vi "Exchange Tool.vi"(8 "error in":errorcluster, 9 "Tool Position":i32, 10 "Place/Pick":enum16{"Place", "Pick"}(ring), 11 "Gantry in":refnum<class "Gantry.lvclass">) -> (0 "error out":errorcluster, 3 "Gantry out":refnum<class "Gantry.lvclass">)   [LabVIEW 2017, in "Gantry.lvclass"]
uses:
  Gantry.lvclass
  Vec3d Class/Vec3d.lvclass
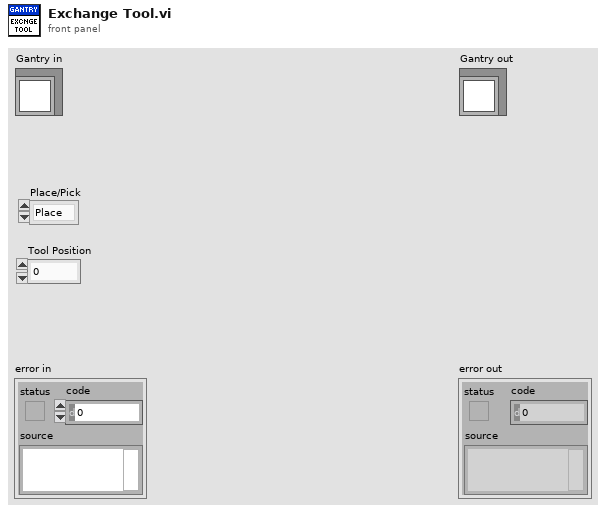
[diagram p1: front panel]
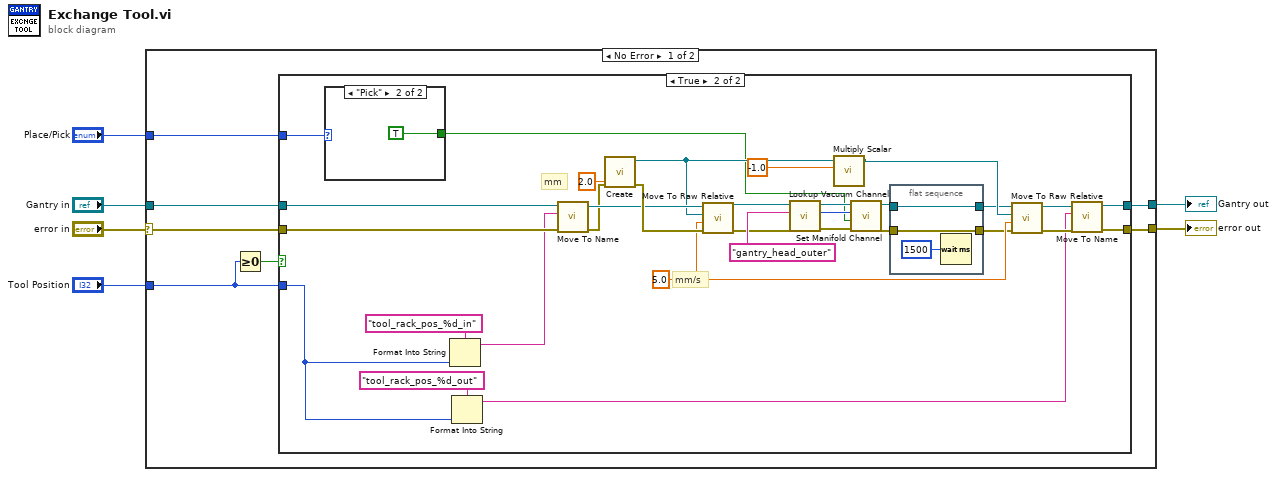
[diagram p0: block diagram]
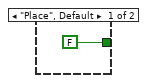
[diagram p3: hidden frame]
diagram:
  n1 = case shown="No Error" "error in" {
    selector: "error in" -> [w10 w52]
    tunnel: "Gantry in" -> [w13 w53]
    tunnel: [w12 w53] -> w5
    tunnel: [w11 w52] -> w3
    tunnel: "Tool Position" -> [w8 _]
    tunnel: "Place/Pick" -> [w9 _]
    frame No Error {
      n2 = Greater Or Equal To 0?(x=w8) -> (x >= 0?=w7:bool)
      n3 = case shown="True" w7 {
        tunnel: w13 -> [w15 w46]
        tunnel: [w15 w45] -> w12
        tunnel: [w14 w44] -> w11
        tunnel: w10 -> [w14 w43]
        tunnel: w9 -> [_ w32]
        tunnel: w8 -> [_ w27]
        frame False {
          # "Specified tool does not live on tool rack (eg syringe)"
        }
        frame True {
          w36 = 5.0 ("Speed")
          # "mm/s"
          # "mm"
          n4 = case shown="\"Pick\"" w32 {
            tunnel: [FALSE TRUE] -> w16
            frame "Place", Default {
            }
            frame "Pick" {
            }
          }
          n5 = Format Into String(format string="tool_rack_pos_%d_in", w27) -> (resulting string=w26:string)  [unwired: 2 in, 1 out]
          n6 = Format Into String(format string="tool_rack_pos_%d_out", w27) -> (resulting string=w25:string)  [unwired: 2 in, 1 out]
          n7 = call-dynamic "Move To Name.vi"("error in"=w43, "Destination"=w26, "Gantry in"=w46) -> ("error out"=w37:errorcluster, "Gantry out"=w38:refnum<class "Gantry.lvclass">)  [unwired: 7 in]
          n8 = call "Create.vi"("error in"=w37, "Z"=2.0) -> ("error out"=w39:errorcluster, "Vec3d Class out"=w35:refnum<class "Vec3d.lvclass">)  [unwired: 8 in]
          n9 = call-dynamic "Move To Raw Relative.vi"("error in"=w39, "Speed(mm/s)"=w36, "Delta"=w35, "Gantry in"=w38) -> ("error out"=w18:errorcluster, "Gantry out"=w17:refnum<class "Gantry.lvclass">)  [unwired: 6 in]
          n10 = call-dynamic "Lookup Vacuum Channel.vi"("error in (no error)"=w18, "Channel Name"="gantry_head_outer", "Gantry Class in"=w17) -> ("error out"=w23:errorcluster, "Channel Number"=w22:i32, "Gantry Class out"=w24:refnum<class "Gantry.lvclass">)  [unwired: 5 in]
          n11 = call-dynamic "Multiply Scalar.vi"("Scale"=-1.0, "Vec3d in"=w35) -> ("Vec3d out"=w33:refnum<class "Vec3d.lvclass">)  [unwired: 8 in, 1 out]
          n12 = call-dynamic "Set Manifold Channel.vi"("error in"=w23, "On/Off"=w16, "Manifold Channel"=w22, "Gantry in"=w24) -> ("error out"=w19:errorcluster, "Gantry out"=w20:refnum<class "Gantry.lvclass">)  [unwired: 6 in]
          n13 = flat-sequence {
            tunnel: w20 -> [w49]
            tunnel: [w49] -> w31
            tunnel: w19 -> [w48]
            tunnel: [w48] -> w30
            frame #0 {
              n14 = Wait (ms)(milliseconds to wait=u32 1500) -> ()  [unwired: 1 out]
            }
          }
          n15 = call-dynamic "Move To Raw Relative.vi"("error in"=w30, "Speed(mm/s)"=w36, "Delta"=w33, "Gantry in"=w31) -> ("error out"=w40:errorcluster, "Gantry out"=w41:refnum<class "Gantry.lvclass">)  [unwired: 6 in]
          n16 = call-dynamic "Move To Name.vi"("error in"=w40, "Destination"=w25, "Gantry in"=w41) -> ("error out"=w44:errorcluster, "Gantry out"=w45:refnum<class "Gantry.lvclass">)  [unwired: 7 in]
        }
      }
    }
    frame Error {
    }
  }
  "error out" <- w3
  "Gantry out" <- w5
